vi "Read.vi"(11 "VolatusApiHttpService in":refnum<class "VolatusApiHttpService.lvclass">) -> (2 "VolatusAPI":refnum<class "VolatusAPI.lvclass">)   [LabVIEW 2020, in "Volatus.lvlib" / "VolatusApiHttpService.lvclass"]
uses:
  VolatusApiHttpService.lvclass
  VolatusApiHttpService.lvclass/VolatusApiHttpService.ctl
  VolatusAPI/VolatusAPI.lvclass
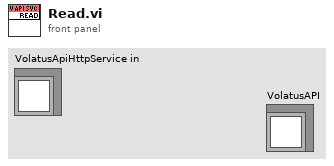
[diagram p1: front panel]
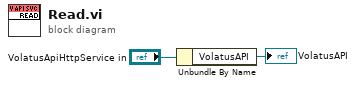
[diagram p0: block diagram]
diagram:
  n1 = Unbundle By Name("VolatusApiHttpService in") -> ("VolatusAPI"=→"VolatusAPI":refnum<class "VolatusAPI.lvclass">)
